vi "Temperature_2.vi"() -> ()   [LabVIEW 2017]
panel:
  in  "Stop Button":bool
  out "Thermometer":dbl(slide) scale=0.0..100.0
  out "Waveform Chart":dbl(graph)
  in  "Slide":dbl(slide) scale=0.0..210.0
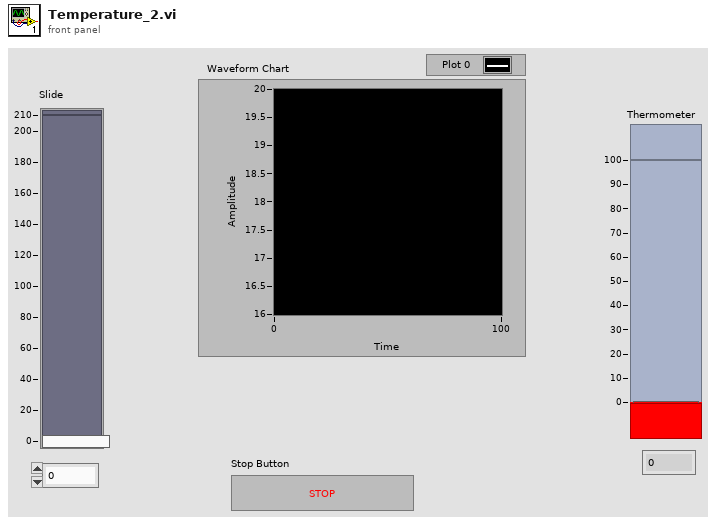
[diagram p1: front panel]
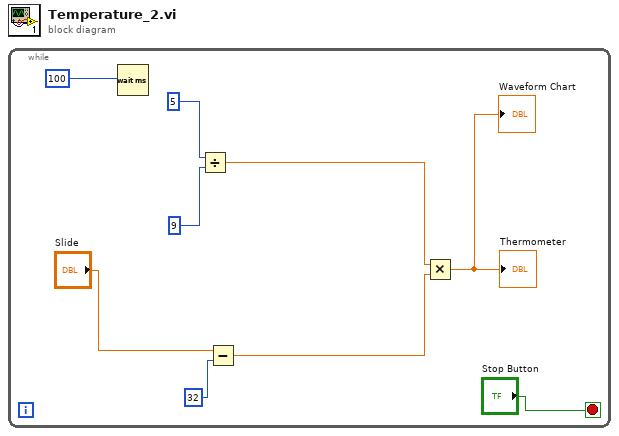
[diagram p0: block diagram]
diagram:
  n1 = while {
    stop <- "Stop Button" stop-if-true
    n2 = Wait (ms)(milliseconds to wait=100) -> ()  [unwired: 1 out]
    n3 = Divide(x=5, y=9) -> (x/y=w5:dbl)
    n4 = Subtract(x="Slide", y=32) -> (x-y=w4:dbl)
    n5 = Multiply(x=w5, y=w4) -> (x*y=→"Waveform Chart" →"Thermometer":dbl)
  }
